vi "Delete Instrument.vi"(8 "error in (no error)":errorcluster, 9 "Tree Tag":string, 11 "Data Cluster":T1) -> (0 "error out":errorcluster, 3 "Data Cluster out":T1)   [LabVIEW 2018, in "Test Manager.lvlib"]
uses:
  Test Manager.lvlib
  Module Data--cluster.ctl
  <vilib>/Delacor/Delacor QMH/Libraries/Message Queue_class/Delacor_lib_QMH_Message Queue.lvclass
  TypeDefs/Comparator Intrument Configuration.ctl
  Mass Cal Measurement Progs/Instrument IO/Cloneable Comparator Drivers/Comparator Classes/Generic/Generic.lvclass
  TypeDefs/Instrument Connection Info.ctl
  Request Events--cluster.ctl
  Stop Argument--cluster.ctl
  Show Panel Argument--cluster.ctl
  Hide Panel Argument--cluster.ctl
  Get Module Execution Status Argument--cluster.ctl
  Show Diagram Argument--cluster.ctl
  Register for Instrument Modules Argument--cluster.ctl
  <vilib>/Delacor/Delacor QMH/Libraries/Message Queue_class/Delacor_lib_QMH_Message Queue.lvclass/Delacor_lib_QMH_Message Queue.ctl
  <vilib>/Delacor/Delacor QMH/Libraries/Message Queue_class/Delacor_lib_QMH_Enqueue Message (Single).vi
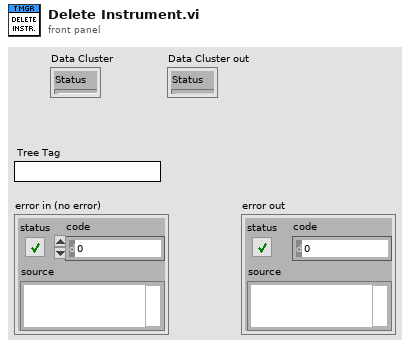
[diagram p1: front panel]
types:
  T1 = typedef "Test Manager.lvlib/Module Data--cluster.ctl" = cluster{"Status":string, "ComparatorPaths":path[], "Comparators":string[], "ThermPaths":path[], "Thermometers":string[], "PressPaths":path[], "PressSensors":string[], "HygroPaths":path[], "Hygrometers":string[], "ComparatorParent":path, "ThermParent":path, "PressParent":path, "HygroParent":path, "Refs":cluster{"Tree":refnum<vi>, "Exit":refnum<vi>, "Name":refnum<vi>, "Channel#":refnum<vi>, "VISA":refnum<vi>}, "Config File":path, "InstConfig":T2[], "Message Queue":refnum<class "Delacor_lib_QMH_Message Queue.lvclass">, "EventRegRef":refnum<event-registration>}
  T2 = typedef "Comparator Intrument Configuration.ctl" = cluster{"Comparator":string, "COM Port":refnum<visa-resource-name>, "Thermometers":T3[], "Hygrometers":T3[], "Barometers":T3[], "Connected?":bool, "CompMod_ID":i16, "Comparator Object":refnum<class "Generic.lvclass">}
  T3 = typedef "Instrument Connection Info.ctl" = cluster{"COM Port":refnum<visa-resource-name>, "Name":string, "Channel #":u16, "Connected?":bool, "Mod_ID":i16}
  T4 = typedef "Test Manager Tree Tag.ctl" = cluster{"ItemType":T5, "VISA Resource":refnum<visa-resource-name>, "Name":string, "Channel #":u16, "ComparatorID":u16}
  T5 = typedef "Tree Item Type.ctl" = enum16{"Comparator", "Temp Group", "Press Group", "Hygro Group", "Thermometer", "PressureTransducer", "Hygrometers", "Add Comparator", "Add Thermometer", "Add Barometer", "Add Hygrometer"}
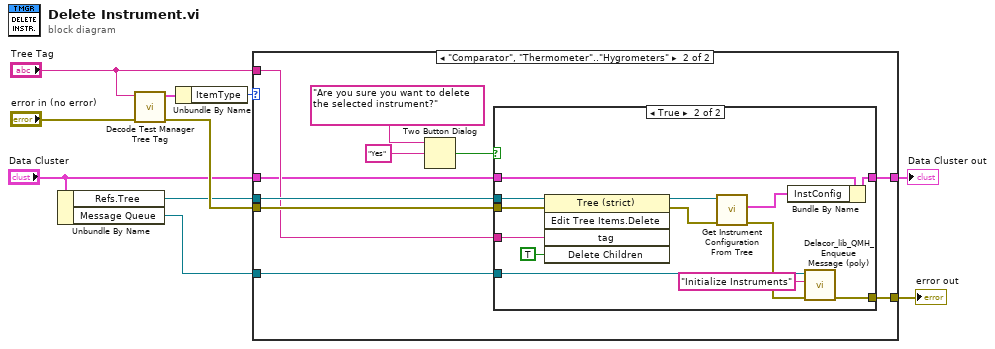
[diagram p0: block diagram]
diagram:
  n1 = Unbundle By Name("Data Cluster") -> ("Refs.Tree"=w4:refnum<vi>, "Message Queue"=w1:refnum<class "Delacor_lib_QMH_Message Queue.lvclass">)
  n2 = call "Decode Test Manager Tree Tag.vi"("error in (no error)"="error in (no error)", "Tag"="Tree Tag") -> ("error out"=w7:errorcluster, "Test Manager Tree Tag"=w9:T4)  [unwired: 8 in]
  n3 = Unbundle By Name(w9) -> ("ItemType"=w10:T5)
  n4 = case shown="\"Comparator\", \"Thermometer\"..\"Hygrometers\"" w10 {
    tunnel: w4 -> [_ w19]
    tunnel: w7 -> [w11 w18]
    tunnel: "Tree Tag" -> [_ w17]
    tunnel: w1 -> [_ w16]
    tunnel: [w11 w15] -> w5
    tunnel: "Data Cluster" -> [w12 w14]
    tunnel: [w12 w13] -> w2
    frame Default {
    }
    frame "Comparator", "Thermometer".."Hygrometers" {
      n5 = Two Button Dialog(message="Are you sure you want to delete the selected instrument?", 2:"Yes" ("T button name (\"OK\")")) -> (T button?=w21:bool)  [unwired: 1 in]
      n6 = case shown="True" w21 {
        tunnel: w19 -> [_ w37]
        tunnel: w18 -> [w23 w36]
        tunnel: w17 -> [_ w35]
        tunnel: w16 -> [_ w33]
        tunnel: [w23 w28] -> w15
        tunnel: w14 -> [w24 w27]
        tunnel: [w24 w26] -> w13
        frame False {
        }
        frame True {
          n7 = invoke class="Tree (strict)" method="Edit Tree Items.Delete"(reference=w37, error in=w36, "tag"=w35, "Delete Children"=TRUE ("Delete Children?")) -> (reference out=w32:refnum<vi>, error out=w31:errorcluster)  [unwired: 1 in, 3 out]
          n8 = call "Get Instrument Configuration From Tree.vi"("error in (no error)"=w31, "Tree ref"=w32) -> ("error out"=w30:errorcluster, "Instrument Config"=w25:T2[])  [unwired: 7 in, 1 out]
          n9 = Bundle By Name(cluster=w27, "InstConfig"=w25) -> (w26:T1)
          n10 = call-poly <vilib>:"Delacor_lib_QMH_Enqueue Message (poly).vi"("error in (no error)"=w30, "Message"="Initialize Instruments", "Message Queue in"=w33) -> ("error out"=w28:errorcluster)  [unwired: 7 in, 1 out]
        }
      }
    }
  }
  "error out" <- w5
  "Data Cluster out" <- w2
